vi "KillPixelsOutsideCircularROI (SubVI).vi"(1 "XY Array":dbl[][](array[numeric]), 2 "Radius*ScaleFactor":dbl, 3 "Center (Pixels)":cluster{"X":sgl, "Y":sgl}) -> (0 "subarray":dbl[][](array[numeric]))   [LabVIEW 2016]
panel:
  out "Modified array":dbl[][](array[numeric])
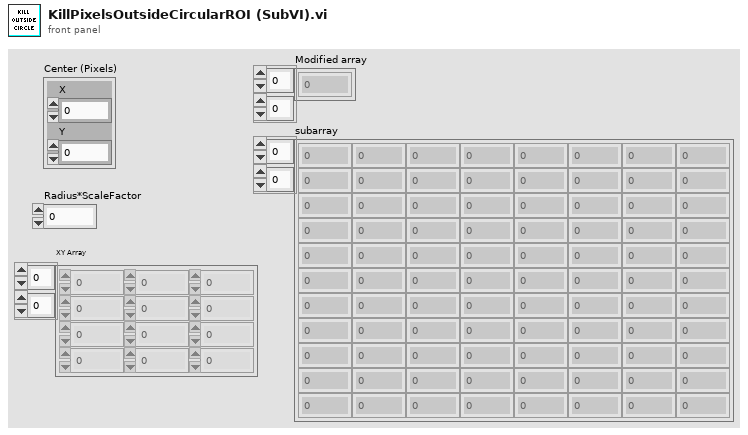
[diagram p1: front panel]
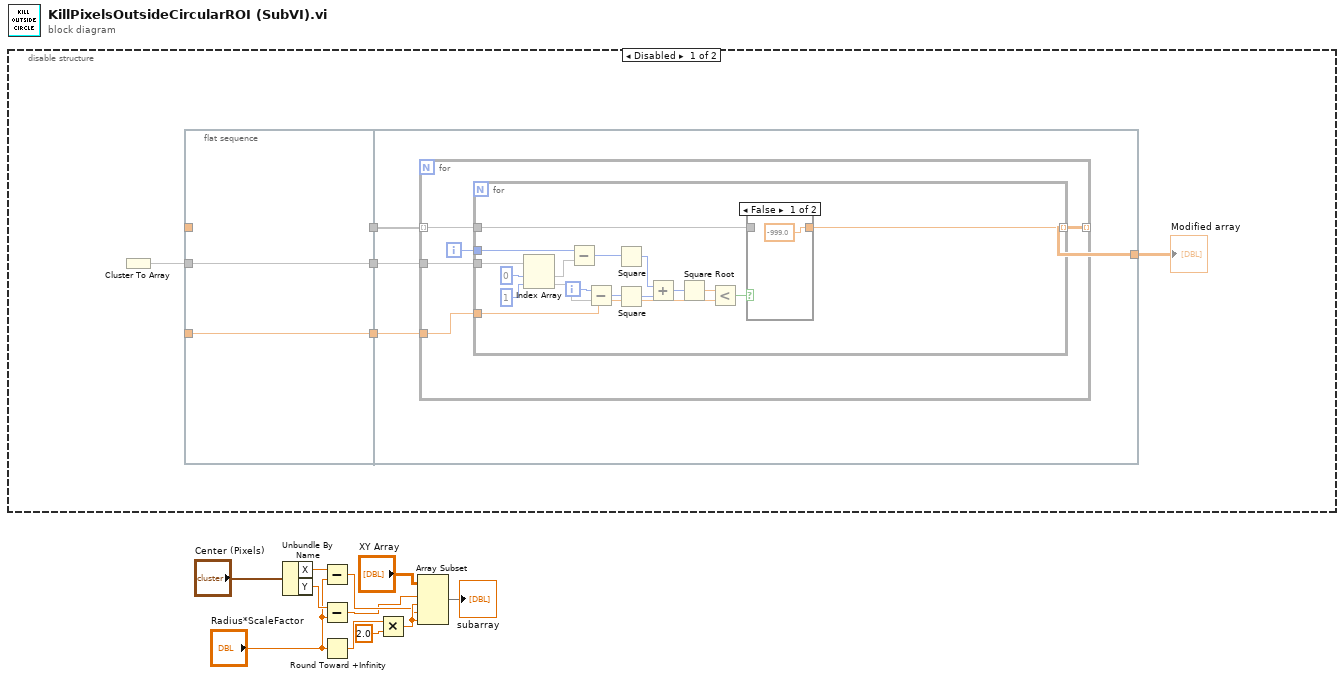
[diagram p0: block diagram]
diagram:
  n1 = disable-structure shown="Disabled" {
    frame Disabled {
      n2 = Cluster To Array() -> (cluster=w15:cluster{void}, array=w14:void[])
      n3 = flat-sequence {
        tunnel: [w22] -> w13
        tunnel: w14 -> [w21]
        tunnel: [_] -> w16
        tunnel: [w20] -> w19
        tunnel: [w21] -> w18
        tunnel: [w22] -> w17
        tunnel: [w23] -> w12
        tunnel: w19 -> [w26]
        tunnel: w18 -> [w25]
        tunnel: w17 -> [w24]
        frame #0 {
        }
        frame #1 {
          n4 = for {
            tunnel: w26 -> [w31] mode=indexing
            tunnel: w25 -> [w29]
            tunnel: w24 -> [w28]
            tunnel: [w27] -> w23 mode=indexing
            i -> [w30]
            n5 = for {
              tunnel: w31 -> [w34]
              tunnel: w29 -> [w46]
              tunnel: w30 -> [w45]
              tunnel: w28 -> [w36]
              tunnel: [w32] -> w27 mode=indexing
              i -> [w41]
              n6 = Index Array(array=w46, index #1=0 ("index"), index #2=1 ("index")) -> (element #1=w44, element #2=w42)
              n7 = Subtract(x=w45, y=w44) -> (x-y=w43:i32)
              n8 = Subtract(x=w41, y=w42) -> (x-y=w40:i32)
              n9 = Square(x=w43) -> (x^2=w39:i32)
              n10 = Square(x=w40) -> (x^2=w38:i32)
              n11 = Add(x=w39, y=w38) -> (x+y=w37:i32)
              n12 = Square Root(x=w37) -> (sqrt(x)=w35:dbl)
              n13 = Less?(x=w35, y=w36) -> (x < y?=w33:bool)
              n14 = case shown="False" w33 {
                tunnel: w34 -> [_ w50]
                tunnel: [-999.0 ("Numeric") w50] -> w32
                frame False {
                }
                frame True {
                }
              }
            }
          }
        }
      }
      "Modified array" <- w12
    }
    frame Enabled {
    }
  }
  n15 = Unbundle By Name("Center (Pixels)") -> ("X"=w10:sgl, "Y"=w9:sgl)
  n16 = Subtract(x=w10, y="Radius*ScaleFactor") -> (x-y=w2:dbl)
  n17 = Subtract(x=w9, y="Radius*ScaleFactor") -> (x-y=w1:dbl)
  n18 = Round Toward +Infinity(x="Radius*ScaleFactor") -> (ceil(x): smallest int >= x=w7:dbl)
  n19 = Multiply(x=w7, y=2.0) -> (x*y=w5:dbl)
  n20 = Array Subset(array="XY Array", index (row)=w1, length (row)=w5, index (col)=w2, length (col)=w5) -> (→"subarray":dbl[][])
